vi "DAQ.Sampling.Coerce Timing.vi"(10 "Max Fs":dbl, 11 "Sampling in":T1 {"Fs" format="%#_13g"}) -> (3 "Sampling out":T1 {"Fs" format="%#_13g"})   [LabVIEW 2019, in "Instrument.Lockin.lvlib" / "Instrument.DAQ.lvclass"]
uses:
  Instrument.DAQ.lvclass
  Typedefs/DAQ.Sampling.Sampling--Cluster.ctl
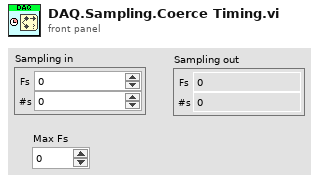
[diagram p1: front panel]
types:
  T1 = typedef "Instrument.Lockin.lvlib/Instrument.DAQ.lvclass/DAQ.Sampling.Sampling--Cluster.ctl" = cluster{"Fs":dbl, "#s":i32}
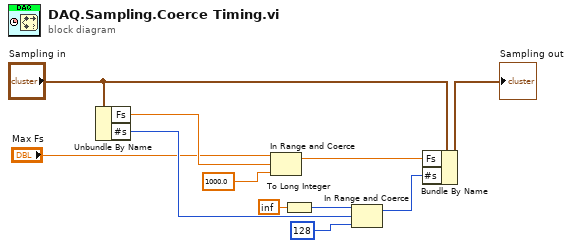
[diagram p0: block diagram]
diagram:
  n1 = Unbundle By Name("Sampling in") -> ("Fs"=w11:dbl, "#s"=w10:i32)
  n2 = In Range and Coerce(upper limit="Max Fs", x=w11, lower limit=1000.0) -> (coerced(x)=w3:dbl)  [unwired: 1 out]
  n3 = To Long Integer(number=inf) -> (32bit integer=w9:i32)
  n4 = In Range and Coerce(upper limit=w9, x=w10, lower limit=128) -> (coerced(x)=w4:i32)  [unwired: 1 out]
  n5 = Bundle By Name(cluster="Sampling in", "Fs"=w3, "#s"=w4) -> (→"Sampling out":T1)
